vi "Set Colour to Table Cell.vi"(9 "Debug Board 2D String":string[][](table), 11 "Debug Board 2D String Ref":refnum<vi>) -> ()   [LabVIEW 2014]
uses:
  <vilib>/Utility/miscctls.llb/LVRowAndColumnTypeDef.ctl
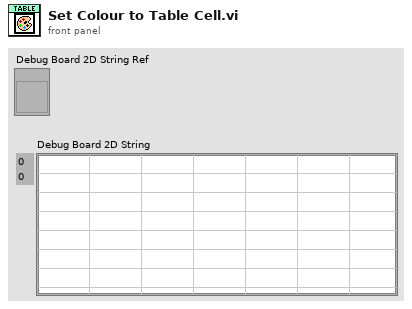
[diagram p1: front panel]
types:
  T1 = typedef "Debug Board 2D String.ctl" = string[][]
  T2 = typedef "LVRowAndColumnTypeDef.ctl" = cluster{"Row":i32, "Column":i32}
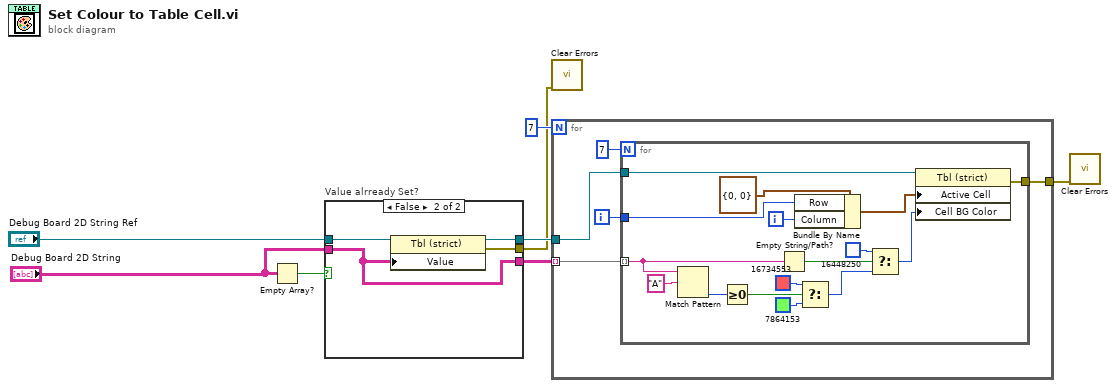
[diagram p0: block diagram]
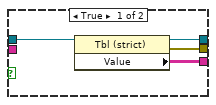
[diagram p2: hidden frame]
diagram:
  n1 = Empty Array?(array="Debug Board 2D String") -> (empty?=w6:bool)
  n2 = case "Value alrready Set?" shown="False" w6 {
    tunnel: "Debug Board 2D String" -> [_ w15]
    tunnel: "Debug Board 2D String Ref" -> [w12 w16]
    tunnel: [w11 w15] -> w1
    tunnel: [w10 w14] -> w3
    tunnel: [w9 w13] -> w2
    frame True {
      n3 = property class="Tbl (strict)"(reference=w12) -> (reference out=w10:refnum<vi>, error out=w9:errorcluster, "Value"=w11:T1)  [unwired: 1 in]
    }
    frame False {
      n4 = property class="Tbl (strict)"(reference=w16, "Value"=w15) -> (reference out=w14:refnum<vi>, error out=w13:errorcluster)  [unwired: 1 in]
    }
  }
  n5 = call <vilib>:"Clear Errors.vi"("error in (no error)"=w2) -> ()  [unwired: 5 in, 2 out]
  n6 = for {
    N: 7 -> [_]
    tunnel: w3 -> [w21]
    tunnel: w1 -> [w18] mode=indexing
    tunnel: [w17] -> w7
    i -> [w19]
    n7 = for {
      N: 7 -> [_]
      tunnel: w21 -> [w37]
      tunnel: w19 -> [w35]
      tunnel: w18 -> [w32] mode=indexing
      tunnel: [w22] -> w17
      i -> [w34]
      n8 = Match Pattern(string=w32, regular expression="A") -> (offset past match=w30:i32)  [unwired: 1 in, 3 out]
      n9 = Greater Or Equal To 0?(x=w30) -> (x >= 0?=w29:bool)
      n10 = Empty String/Path?(string/path=w32) -> (empty?=w26:bool)
      n11 = Bundle By Name(cluster=T2 {"Row"=0, "Column"=0} ("Active Cell:Active Cell"), "Row"=w35, "Column"=w34) -> (w33:T2)
      n12 = Select(t=u32 16734553 ("Color Box"), s=w29, f=u32 7864153 ("Color Box")) -> (s? t:f=w25:u32)
      n13 = Select(t=u32 16448250 ("Color Box"), s=w26, f=w25) -> (s? t:f=w24:u32)
      n14 = property class="Tbl (strict)"(reference=w37, "Active Cell"=w33, "Cell BG Color"=w24) -> (error out=w22:errorcluster)  [unwired: 1 in, 1 out]
    }
  }
  n15 = call <vilib>:"Clear Errors.vi"("error in (no error)"=w7) -> ()  [unwired: 5 in, 2 out]
